vi "Encoder_daq.vi"() -> ()   [LabVIEW 2026]
uses:
  <vilib>/Instr/_visa.llb/VISA Configure Serial Port (Instr).vi
panel:
  out "concatenated string":string
  in  "data bits (8)":u16=8 min=5 max=8 step=1
  out "data":dynamicdata(graph)
  out "read buffer":string
  out "Scalar":dbl
  out "PWM":dbl
  out "Waveform Chart":cluster{"Scalar":dbl, dbl}(graph)
  in  "baud rate (9600)":u32=9600
  in  "VISA resource name":refnum<visa-resource-name>
  in  "stop":bool
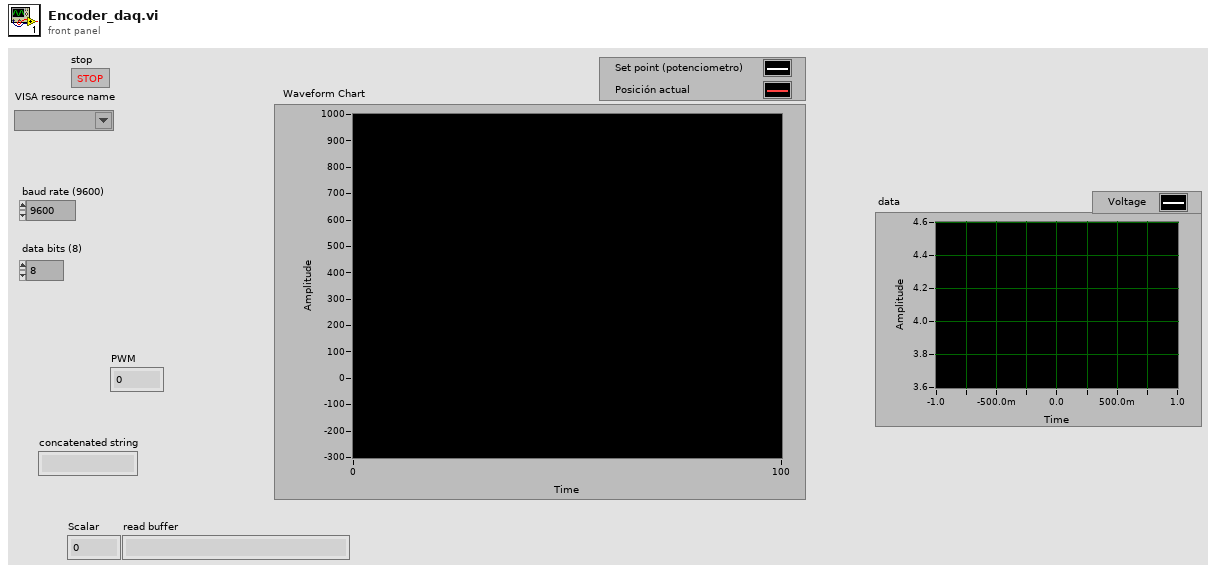
[diagram p1: front panel]
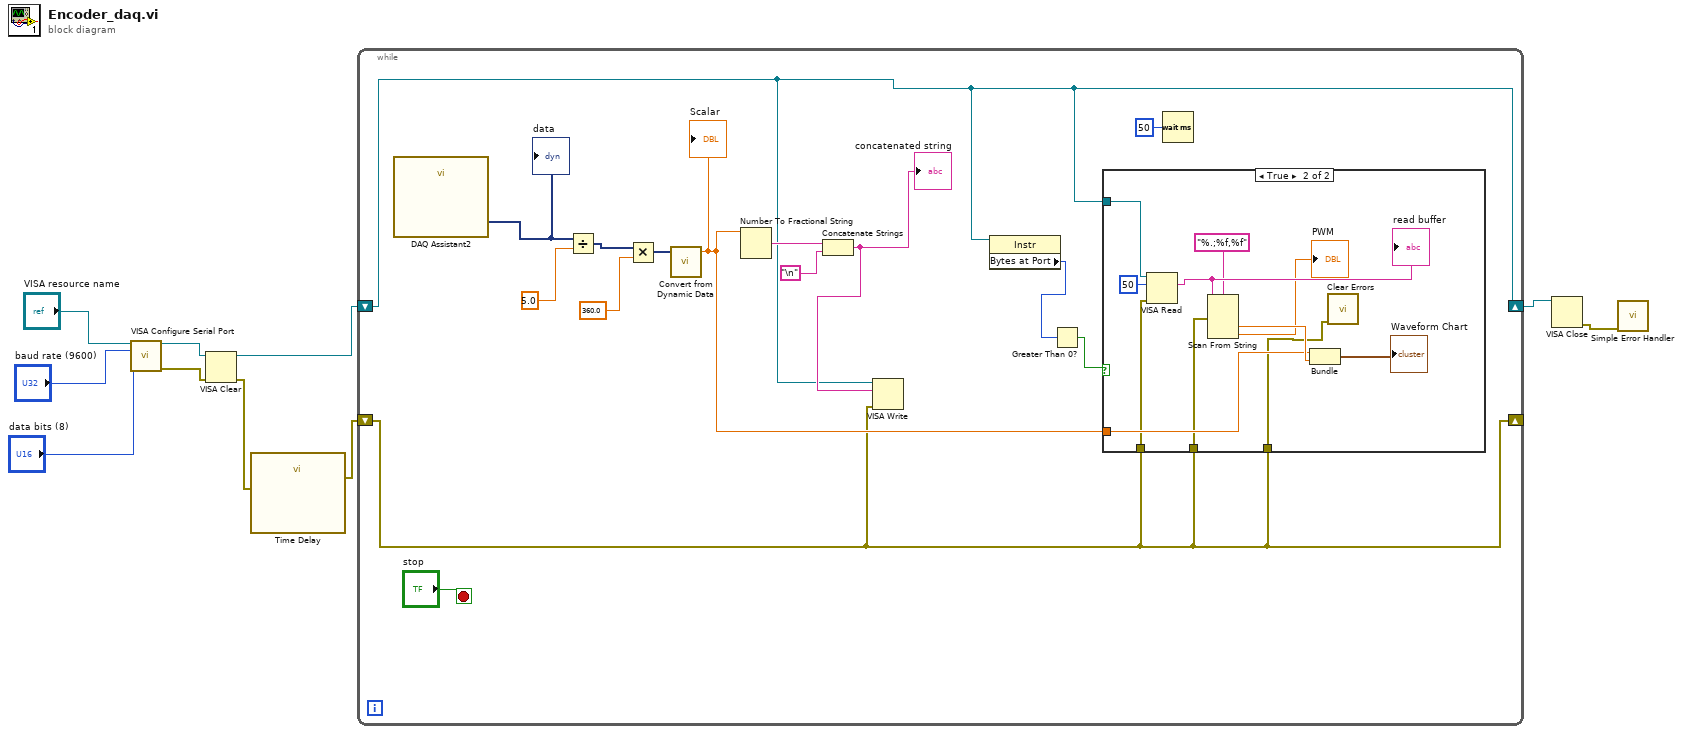
[diagram p0: block diagram]
diagram:
  n1 = call-poly "VISA Configure Serial Port"("VISA resource name"="VISA resource name", "baud rate (9600)"="baud rate (9600)", "data bits (8)"="data bits (8)") -> ("VISA resource name out"=w5:refnum<visa-resource-name>, "error out"=w4:errorcluster)  [unwired: 11 in]
  n2 = VISA Clear(VISA resource name=w5, error in (no error)=w4) -> (VISA resource name out=w3:refnum<visa-resource-name>, error out=w2:errorcluster)
  n3 = call "Time Delay"("error in (no error)"=w2) -> ("error out"=w1:errorcluster)  [unwired: 10 in]
  n4 = while {
    shift-right: [w12] -> w9
    shift-left: w3 -> [w12]
    shift-right: [w11] -> _
    shift-left: w1 -> [w11]
    stop <- "stop" stop-if-true
    n5 = call "DAQ Assistant2"() -> ("data"=w13:dynamicdata)  [unwired: 17 in, 2 out]
    "data" <- w13
    n6 = Divide(x=w13, y=5.0) -> (x/y=w23:dynamicdata)
    n7 = Multiply(x=w23, y=360.0) -> (x*y=w16:dynamicdata)
    n8 = call "Convert from Dynamic Data"("Dynamic Data Type"=w16) -> ("Scalar"=w17:dbl)  [unwired: 3 in]
    "Scalar" <- w17
    n9 = Number To Fractional String(number=w17) -> (F-format string=w21:string)  [unwired: 3 in]
    n10 = Concatenate Strings(w21, "\n") -> (w19:string)
    "concatenated string" <- w19
    n11 = VISA Write(VISA resource name=w12, write buffer=w19, error in (no error)=w11) -> ()  [unwired: 3 out]
    n12 = property class="Instr"(reference=w12) -> ("Bytes at Port"=w15:u32)  [unwired: 1 in, 2 out]
    n13 = Greater Than 0?(x=w15) -> (x > 0?=w14:bool)
    n14 = case shown="True" w14 {
      tunnel: w17 -> [_ w31]
      tunnel: w12 -> [_ w29]
      tunnel: w11 -> [_ w28]
      tunnel: w11 -> [_ w27]
      tunnel: w11 -> [_ w26]
      frame False {
      }
      frame True {
        n15 = VISA Read(VISA resource name=w29, byte count=u32 50, error in (no error)=w28) -> (read buffer=w36:string)  [unwired: 3 out]
        "read buffer" <- w36
        n16 = Scan From String "Scan From String"(format string="%.;%f,%f", input string=w36, error in=w27) -> (output 1=w34:dbl, output 2=→"PWM":dbl)  [unwired: 3 in, 3 out]
        n17 = Bundle("Scalar"=w31, w34) -> (→"Waveform Chart":cluster{"Scalar":dbl, dbl})  [unwired: 1 in]
        n18 = call <vilib>:"Clear Errors.vi"("error in (no error)"=w26) -> ()  [unwired: 5 in, 2 out]
      }
    }
    n19 = Wait (ms)(milliseconds to wait=u32 50) -> ()  [unwired: 1 out]
  }
  n20 = VISA Close(VISA resource name=w9) -> (error out=w8:errorcluster)  [unwired: 1 in]
  n21 = call <vilib>:"Simple Error Handler.vi"("error in (no error)"=w8) -> ()  [unwired: 4 in, 5 out]
